vi "Load Script.vi"(7 "Script Name":string="TSB_Script", 8 "error in (no error)":errorcluster caption="错误输入（无错误）", 10 "Script":string, 11 "虚拟 输入":refnum<class "虚拟.lvclass">) -> (0 "error out":errorcluster caption="错误输出", 3 "虚拟 输出":refnum<class "虚拟.lvclass">)   [LabVIEW 2020, in "虚拟.lvclass"]
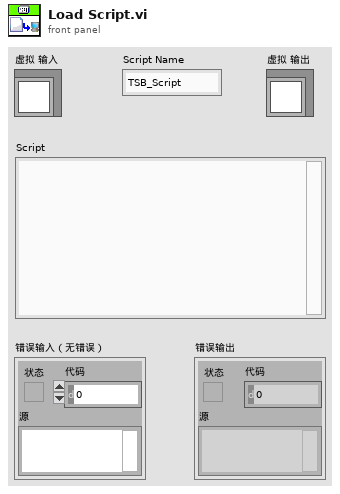
[diagram p1: front panel]
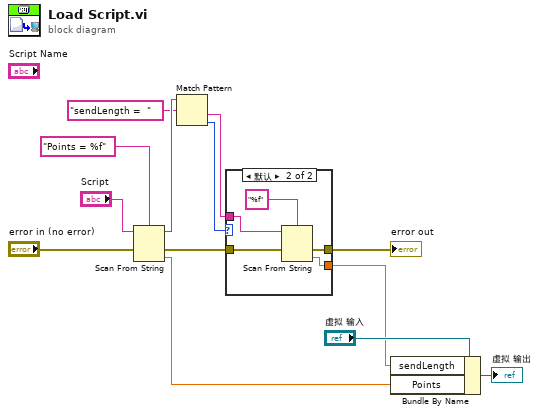
[diagram p0: block diagram]
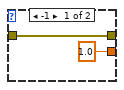
[diagram p2: hidden frame]
diagram:
  n1 = Scan From String(format string="Points = %f" ("格式字符串"), input string="Script", error in="error in (no error)") -> (remaining string=w11:string, error out=w3:errorcluster, output 1=w1:dbl)  [unwired: 2 in, 1 out]
  n2 = Match Pattern(string=w11, regular expression="sendLength =  " ("正则表达式")) -> (after substring=w9:string, offset past match=w8:i32)  [unwired: 1 in, 2 out]
  n3 = case shown="默认" w8 {
    tunnel: w9 -> [_ w20]
    tunnel: [1.0 w18] -> w6
    tunnel: w3 -> [w14 w17]
    tunnel: [w14 w16] -> w2
    frame -1 {
    }
    frame Default {
      n4 = Scan From String(format string="%f" ("格式字符串"), input string=w20, error in=w17) -> (error out=w16:errorcluster, output 1=w18:dbl)  [unwired: 2 in, 2 out]
    }
  }
  "error out" <- w2
  n5 = Bundle By Name(cluster="虚拟 输入", "sendLength"=w6, "Points"=w1) -> (→"虚拟 输出":refnum<class "虚拟.lvclass">)
